vi "path.vi"(9 "Wybierz plik:":path) -> (0 "Cancel?":bool, 2 "ród³o 2":path)   [LabVIEW 2023]
panel:
  in  "Cancel Button":bool
  in  "OK Button":bool
  # "Zapisz jako:"
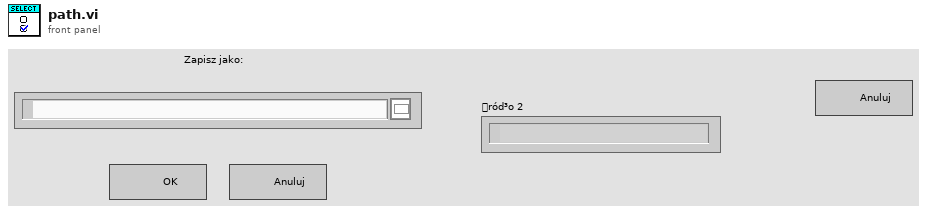
[diagram p1: front panel]
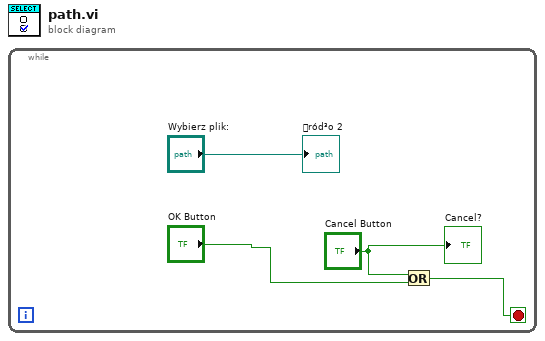
[diagram p0: block diagram]
diagram:
  n1 = while {
    stop <- w1 stop-if-true
    n2 = Or(x="Cancel Button", y="OK Button") -> (x .or. y?=w1:bool)
    "ród³o 2" <- "Wybierz plik:"
    "Cancel?" <- "Cancel Button"
  }
